vi "Create Client Context.vi"(8 "error in (no error)":errorcluster) -> (0 "error out":errorcluster, 3 "ContextID out":T1)   [LabVIEW 2019, in "grpc-lvsupport.lvlib"]
uses:
  grpc-lvsupport.lvlib
  grpcId.ctl
  <vilib>/Utility/error.llb/Error Cluster From Error Code.vi
  <resource>/labview_grpc_server.dll
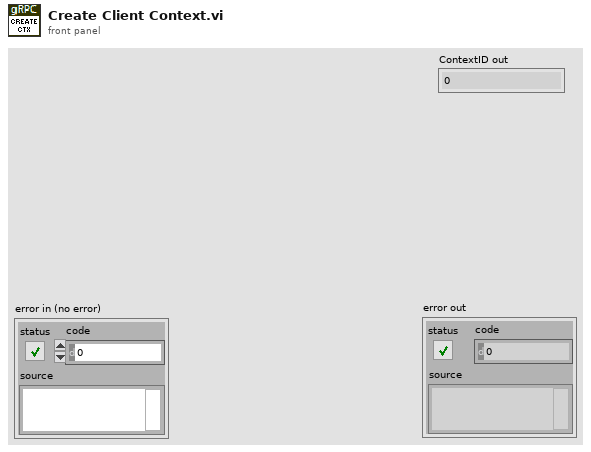
[diagram p1: front panel]
types:
  T1 = typedef "grpc-lvsupport.lvlib/grpcId.ctl" = u64
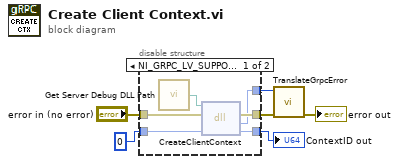
[diagram p0: block diagram]
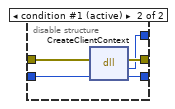
[diagram p2: hidden frame]
diagram:
  n1 = disable-structure shown="NI_GRPC_LV_SUPPORT_DEBUG==True&&RUN_TIME_ENGINE==False" {
    disable-tunnel: "error in (no error)" -> [w11 w17]
    disable-tunnel: [w10 w16] -> w5
    disable-tunnel: [w9 w15] -> w4
    disable-tunnel: [w8 w14] -> w3
    disable-tunnel: u64 0 ("contextId") -> [w7 w13]
    frame condition #0 {
      n2 = call "Get Server Debug DLL Path.vi"() -> ("DLL Path"=w12:path)
      n3 = dll-call lib="?" fn="CreateClientContext"(path in=w12, error in=w11, "contextId"=w7) -> (error out=w9:errorcluster, "return type"=w8:i32, "contextId"=w10:u64)  [unwired: 1 in, 1 out]
    }
    frame condition #1 (active) {
      n4 = dll-call lib="C:/Program Files (x86)/National Instruments/LabVIEW 2024/resource/labview_grpc_server.*" fn="CreateClientContext"(error in=w17, "contextId"=w13) -> (error out=w15:errorcluster, "return type"=w14:i32, "contextId"=w16:u64)  [unwired: 2 in, 1 out]
    }
  }
  "ContextID out" <- w5
  n5 = call "TranslateGrpcError.vi"("error in"=w4, "Error Code"=w3) -> ("error out"=→"error out":errorcluster)  [unwired: 9 in]
